vi "QTMCommanderTEST.vi"(4 "Error In":errorcluster) -> ()   [LabVIEW 2017]
uses:
  <userlib>/QLC/QLC.lvlib
panel:
  out "result":bool
  in  "stop":bool
  out "Numeric 2":i32
  out "LoopTime 2":u32(graph)
  out "LoopTime":u32(graph)
  out "Numeric":i32
  in  "Send Trig":bool
  in  "Stop Capture":bool
  in  "Close Measurement":bool
  in  "New Measurement":bool caption="Start Measurement"
  in  "Start Capture":bool
  out "Camera Timestamp":u64
  out "Camera Frame Num":u32
  out "Controlling QTM":bool
  out "Last QTM Event":dbl=2.0
  out "QTM Message":string
  # "Qualisys Commander"
  # "Qualisys commands"
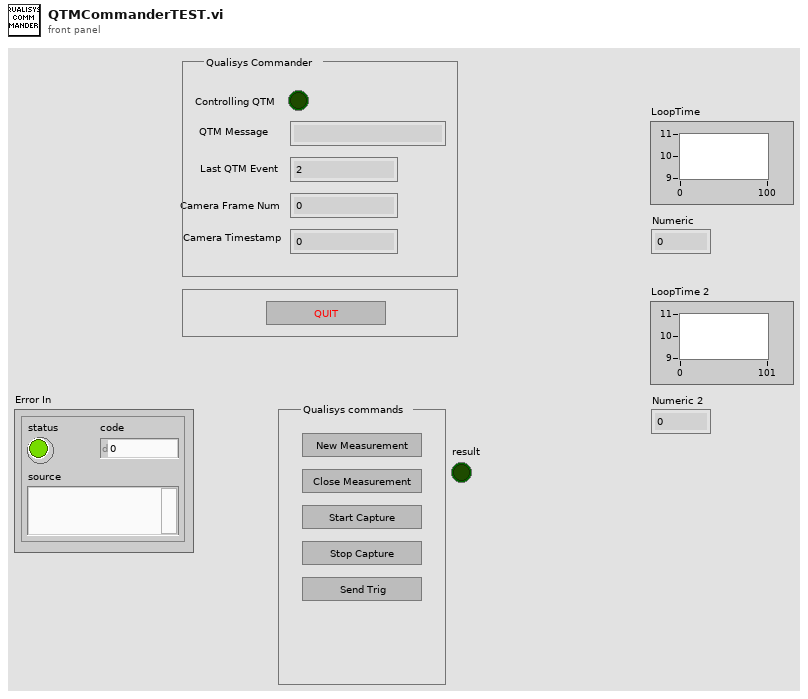
[diagram p1: front panel]
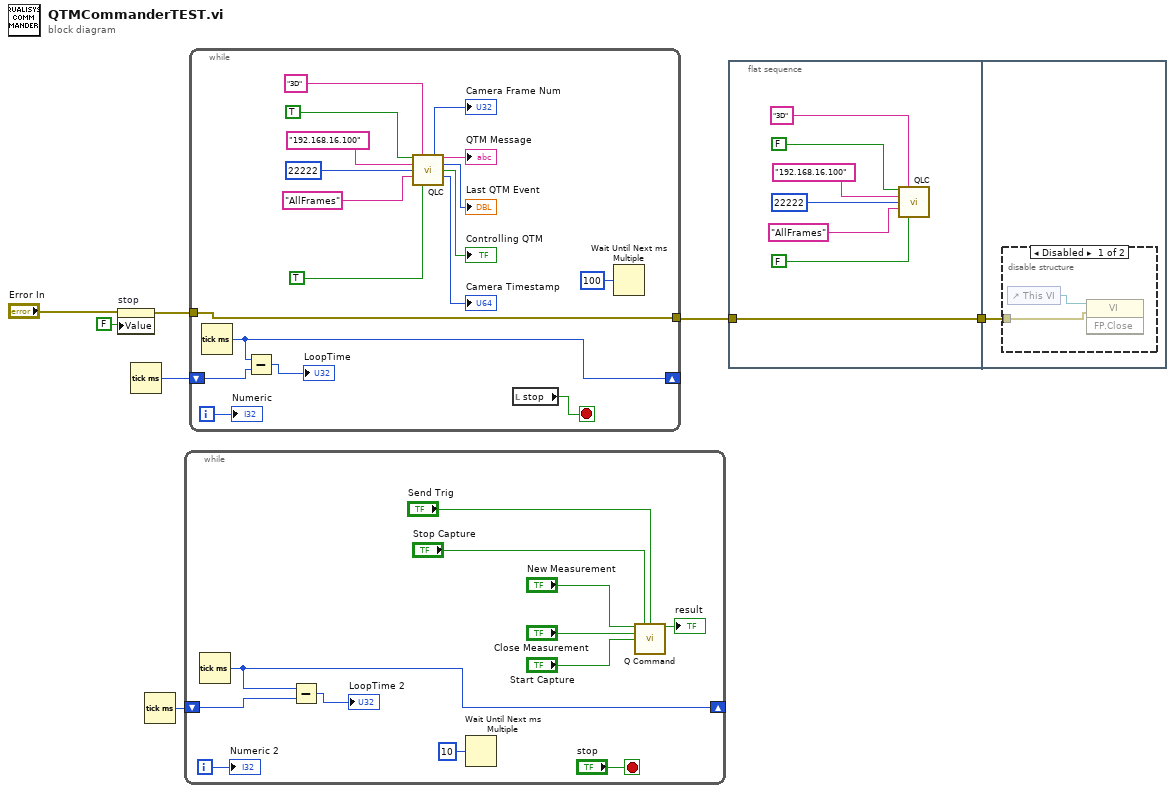
[diagram p0: block diagram]
diagram:
  n1 = property on="stop" class="Bool (strict)"(error in="Error In", "Value"=FALSE ("stop")) -> (error out=w6:errorcluster)  [unwired: 1 in, 1 out]
  n2 = Tick Count (ms)() -> (millisecond timer value=w7:u32)
  n3 = Tick Count (ms)() -> (millisecond timer value=w1:u32)
  n4 = while {
    shift-right: [w16] -> _
    shift-left: w1 -> [w17]
    i -> [w18]
    stop <- "stop" stop-if-true
    n5 = Tick Count (ms)() -> (millisecond timer value=w16:u32)
    n6 = Subtract(x=w16, y=w17) -> (x-y=→"LoopTime 2":u32)
    n7 = Wait Until Next ms Multiple(millisecond multiple=u32 10) -> ()  [unwired: 1 out]
    n8 = call <userlib>:"Q Command.vi"("bNew"="New Measurement", "bStop"="Stop Capture", "bTrig"="Send Trig", "bClose"="Close Measurement", "bStart"="Start Capture") -> ("result"=→"result":bool)  [unwired: 10 in]
    "Numeric 2" <- w18
  }
  n9 = while {
    shift-right: [w24] -> _
    shift-left: w7 -> [w25]
    tunnel: w6 -> [w20]
    tunnel: [w20] -> w3
    i -> [w26]
    stop <- w21 stop-if-true
    n10 = Tick Count (ms)() -> (millisecond timer value=w24:u32)
    n11 = Subtract(x=w24, y=w25) -> (x-y=→"LoopTime":u32)
    n12 = call <userlib>:"QLC.vi"("connect"=TRUE ("Connect to QTM"), "data"="3D" ("Data"), "address"="192.168.16.100" ("Address"), "port"=22222 ("Port"), "frequency"="AllFrames" ("Frequency"), "controlQTM"=TRUE ("Control QTM")) -> ("camFrameNumber"=→"Camera Frame Num":u32, "message"=→"QTM Message":string, "lastEvent"=→"Last QTM Event":i32, "QTMMaster"=→"Controlling QTM":bool, "camTimeStamp"=→"Camera Timestamp":u64)  [unwired: 4 in, 1 out]
    n13 = local read "stop"() -> (w21:bool)
    n14 = Wait Until Next ms Multiple(millisecond multiple=u32 100) -> ()  [unwired: 1 out]
    "Numeric" <- w26
  }
  n15 = flat-sequence {
    tunnel: w3 -> [w44]
    tunnel: [w44] -> w2
    tunnel: w2 -> [w45]
    frame #0 {
      n16 = call <userlib>:"QLC.vi"("connect"=FALSE ("Connect to QTM"), "data"="3D" ("Data"), "address"="192.168.16.100" ("Address"), "port"=22222 ("Port"), "frequency"="AllFrames" ("Frequency"), "controlQTM"=FALSE ("Control QTM")) -> ()  [unwired: 4 in, 6 out]
    }
    frame #1 {
      n17 = disable-structure shown="Disabled" {
        disable-tunnel: w45 -> [w46 _]
        frame Disabled {
          n18 = control-ref of="This VI"() -> (w47:refnum<vi>)
          n19 = invoke class="VI" method="FP.Close"(reference=w47, error in=w46) -> ()  [unwired: 1 in, 3 out]
        }
        frame Enabled {
        }
      }
    }
  }
